vi "Module.Reset Children.vi"(11 "Child Modules":cluster{"Name":string, "vi ref":refnum<vi>}[](array[cluster])) -> ()   [LabVIEW 2018]
uses:
  <vilib>/KATE/Queues/Queue Utils.lvlib
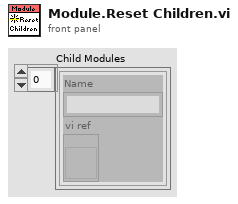
[diagram p1: front panel]
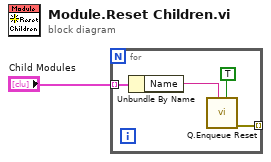
[diagram p0: block diagram]
diagram:
  n1 = for {
    tunnel: "Child Modules" -> [w5] mode=indexing
    tunnel: [w3] -> _ mode=indexing
    n2 = Unbundle By Name(w5) -> ("Name"=w4:string)
    n3 = call <vilib>:"Q.Enqueue Reset.vi"("Top of Q(T)"=TRUE, "Q Name"=w4) -> ("error out"=w3:errorcluster)  [unwired: 8 in, 1 out]
  }
